vi "Main.vi"() -> ()   [LabVIEW 2019]
uses:
  <vilib>/sound2/lvsound2.llb/Sound Data Format.ctl
  <vilib>/sound2/lvsound2.llb/Sampling Mode.ctl
  <vilib>/sound2/lvsound2.llb/Sound Input Read (DBL).vi
panel:
  out "Raw Data":waveform(dbl)[](graph)
  out "Spectrum Data":cluster{"f0":dbl, "df":dbl, "magnitude":dbl[]}[](graph)
  out "Threshold Exceeded?":bool
  in  "Threshold, dB":dbl=-100.0 format="%#_13g"
  in  "Upper Fc":dbl=3500.0 format="%#_13g"
  in  "Lower Fc":dbl=300.0 format="%#_13g"
  in  "Order":i32=6
  in  "Type":T1(ring)
  in  "Stop":bool
  # "FILTER SETTINGS"
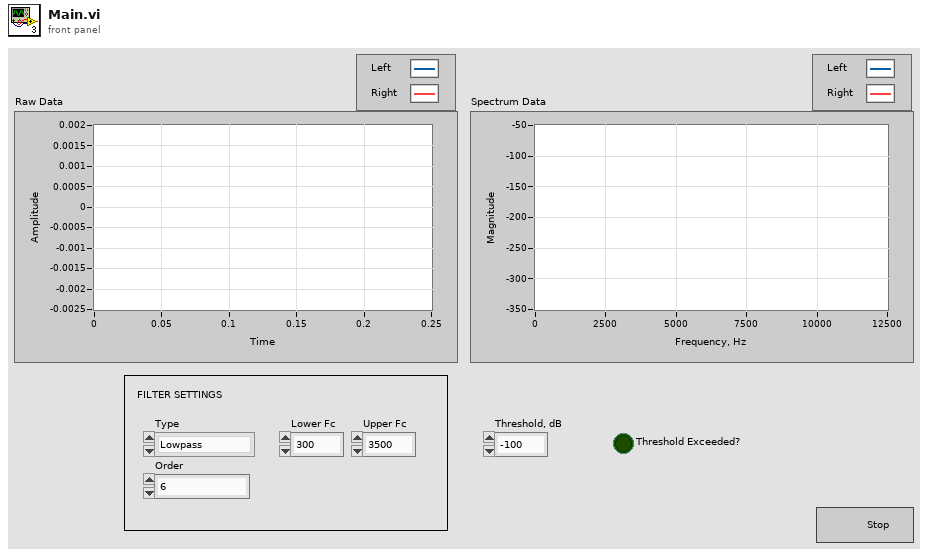
[diagram p1: front panel]
types:
  T1 = enum16{"Lowpass", "Highpass", "Bandpass", "Bandstop"}
  T2 = typedef "Sampling Mode.ctl" = i32
  T3 = typedef "Sound Data Format.ctl" = cluster{"sample rate (S/s)":dbl, "number of channels":i32, "bits per sample":i32}
  T4 = typedef "Sound Input Task ID.ctl" = u32
  T5 = cluster{"Topology":enum16{"Off", "Butterworth", "Chebyshev", "Inverse Chebyshev", "Elliptic", "Bessel"}, "Type":enum16{"Lowpass", "Highpass", "Bandpass", "Bandstop"}, "Order":i32, "Lower Fc":dbl, "Upper Fc":dbl, "PB Ripple":dbl, "SB Attenuation":dbl}
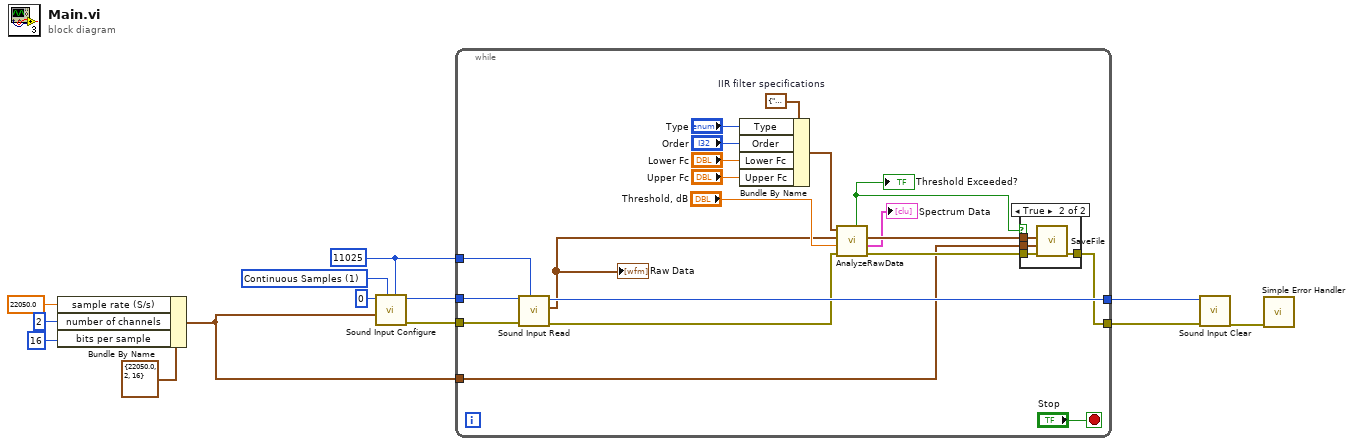
[diagram p0: block diagram]
diagram:
  w1 = 11025 ("Number of Samples/ch")
  w7 = T2 1 items=["Finite Samples", "Continuous Samples"] ("sample mode")
  n1 = Bundle By Name(cluster=T3 {"sample rate (S/s)"=22050.0, "number of channels"=2, "bits per sample"=16} ("sound format"), "sample rate (S/s)"=22050.0 ("Sample rate (Hz)"), "number of channels"=2 ("#Channels"), "bits per sample"=16 ("Resolution (bits)")) -> (w5:T3)
  n2 = call <vilib>:"Sound Input Configure.vi"("number of samples/ch"=w1, "sample mode"=w7, "sound format"=w5, "device ID"=u32 0 ("Device")) -> ("error out"=w13:errorcluster, "task ID"=w6:T4)  [unwired: 6 in]
  n3 = while {
    tunnel: w13 -> [w33]
    tunnel: w6 -> [w32]
    tunnel: w1 -> [w31]
    tunnel: w5 -> [w15]
    tunnel: [w16] -> w4
    tunnel: [w25] -> w2
    stop <- "Stop" stop-if-true
    w30 = T5 {"Topology"=enum."Butterworth", "Type"=enum."Lowpass", "Order"=1, "Lower Fc"=100.0, "Upper Fc"=200.0, "PB Ripple"=1.0, "SB Attenuation"=60.0}  # IIR filter specifications
    n4 = call-poly <vilib>:"Sound Input Read.vi"("number of samples/ch"=w31, "error in (no error)"=w33, "task ID"=w32) -> ("error out"=w23:errorcluster, "data"=w21:waveform(dbl)[], "task ID out"=w25:T4)  [unwired: 6 in]
    "Raw Data" <- w21
    n5 = Bundle By Name(cluster=w30, "Type"="Type", "Order"="Order", "Lower Fc"="Lower Fc", "Upper Fc"="Upper Fc") -> (w20:T5)
    n6 = call "AnalyzeRawData.vi"("error in (no error)"=w23, "Threshold, dB"="Threshold, dB", "Raw Data"=w21, "IIR Filter Specifications"=w20) -> ("error out"=w17:errorcluster, "Power Spectrum / PSD"=→"Spectrum Data":cluster{"f0":dbl, "df":dbl, "magnitude":dbl[]}[], "Filtered Data"=w19:waveform(dbl)[], "Threshold Exceeded?"=w14:bool)  [unwired: 4 in]
    "Threshold Exceeded?" <- w14
    n7 = case shown="True" w14 {
      tunnel: w19 -> [_ w38]
      tunnel: w17 -> [w34 w37]
      tunnel: [w34 w36] -> w16
      tunnel: w15 -> [_ w35]
      frame False {
      }
      frame True {
        n8 = call "SaveFile.vi"("error in (no error)"=w37, "sound format"=w35, "Filtered Data"=w38) -> ("error out"=w36:errorcluster)  [unwired: 7 in, 1 out]
      }
    }
  }
  n9 = call <vilib>:"Sound Input Clear.vi"("error in (no error)"=w4, "task ID"=w2) -> ("error out"=w3:errorcluster)  [unwired: 9 in]
  n10 = call <vilib>:"Simple Error Handler.vi"("error in (no error)"=w3) -> ()  [unwired: 4 in, 5 out]
